vi "fgt get valve Channel Count.vi"(8 "error in (no error)":errorcluster) -> (0 "error out":errorcluster, 3 "nbVChan out":u32)   [LabVIEW 2016, in "fgt_SDK.lvlib"]
doc: "Get total number of initialized valve channels.\n\nIt is the sum of all connected Two-Switch, L-Switch and M-Switch valves connected to Switchboard or Switch EZ devices, as well as individual P-Switch outputs (8 per device)."
uses:
  fgt_SDK.lvlib
  dlls/fgt_SDK_32.dll
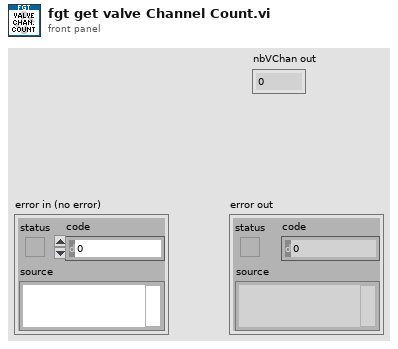
[diagram p1: front panel]
types:
  T1 = typedef "fgt_SDK.lvlib/fgt_STATUS_INFO.ctl" = cluster{"InstrType":T2, "instrSN":u16, "errorCode":u8, "infoCode":u8, "detail":string}
  T2 = typedef "fgt_SDK.lvlib/fgt_INSTRUMENT_TYPE.ctl" = enum32{"None", "MFCS", "MFCS_EZ", "FRP", "LineUP", "IPS"}
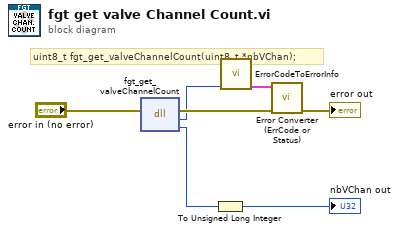
[diagram p0: block diagram]
diagram:
  # "uint8_t fgt_get_valveChannelCount(uint8_t *nbVChan);"
  n1 = dll-call lib="C:/projects/SDK/fgt-sdk-labview/dlls/fgt_SDK_*.*" fn="fgt_get_valveChannelCount"(error in="error in (no error)") -> (error out=w6:errorcluster, "return type"=w4:u8, "nbVChan"=w2:u8)  [unwired: 3 in, 1 out]
  n2 = To Unsigned Long Integer(number=w2) -> (unsigned 32bit integer=→"nbVChan out":u32)
  n3 = call "ErrorCodeToErrorInfo.vi"("return type"=w4) -> ("StatusInfo"=w3:T1)  [unwired: 10 in]
  n4 = call "Error Converter (ErrCode or Status).vi"("error in (no error)"=w6, "StatusInfo"=w3) -> ("error out"=→"error out":errorcluster)  [unwired: 9 in]
